vi "DataLogger_CloseFile.vi"(8 "error in (no error)":errorcluster, 11 "Data Logger in":refnum<class "Data Logger.lvclass">) -> (0 "error out":errorcluster, 3 "Data Logger out":refnum<class "Data Logger.lvclass">)   [LabVIEW 2016, in "Data Logger.lvclass"]
uses:
  Data Logger.lvclass
  Data Logger.lvclass/Data Logger.ctl
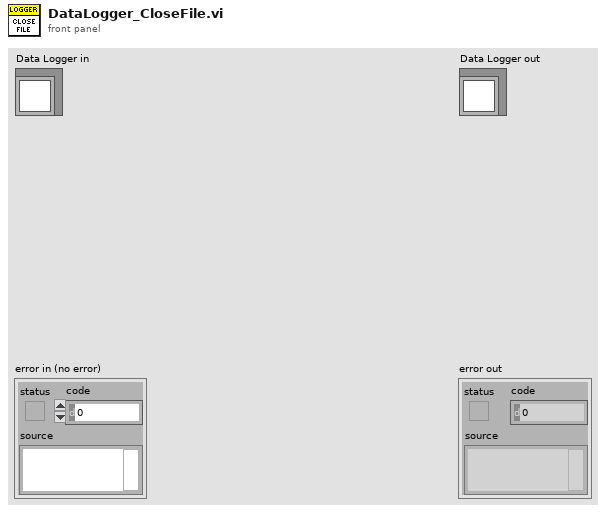
[diagram p1: front panel]
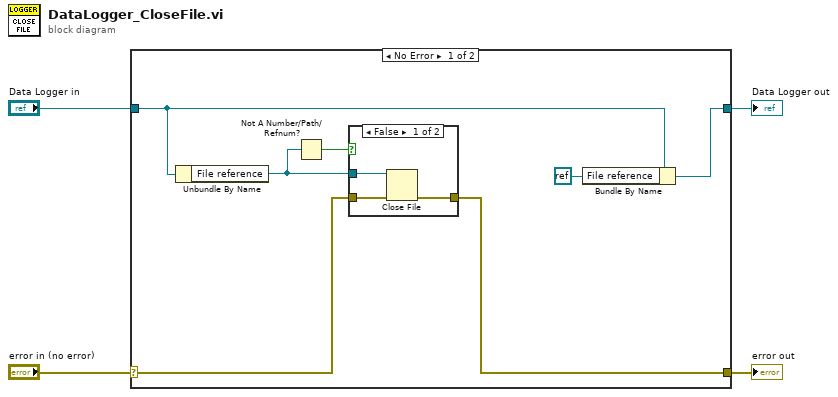
[diagram p0: block diagram]
diagram:
  n1 = case shown="No Error" "error in (no error)" {
    selector: "error in (no error)" -> [w9 w17]
    tunnel: [w8 w17] -> w3
    tunnel: [w6 w16] -> w1
    tunnel: "Data Logger in" -> [w7 w16]
    frame No Error {
      n2 = Unbundle By Name(w7) -> ("File reference"=w10:refnum<file>)
      n3 = Not A Number/Path/Refnum?(number/path/refnum=w10) -> (NaN/Path/Refnum?=w11:bool)
      n4 = case shown="False" w11 {
        tunnel: w9 -> [w14 w15]
        tunnel: [w13 w15] -> w8
        tunnel: w10 -> [w12 _]
        frame False {
          n5 = Close File(refnum=w12, error in=w14) -> (error out=w13:errorcluster)  [unwired: 1 out]
        }
        frame True {
        }
      }
      n6 = Bundle By Name(cluster=w7, "File reference"=refnum<k0> refnum) -> (w6:refnum<class "Data Logger.lvclass">)
    }
    frame Error {
    }
  }
  "error out" <- w3
  "Data Logger out" <- w1
